vi "Set IC.vi"(8 "error in (no error)":errorcluster, 10 "IC":variant, 11 "IC in":refnum<class "NI_IC.lvclass">) -> (0 "error out":errorcluster, 3 "IC out":refnum<class "NI_IC.lvclass">)   [LabVIEW 2020, in "NI_PDE.lvlib" / "NI_IC.lvclass"]
uses:
  <vilib>/gmath/pde.llb/ICClass/NI_IC.lvclass
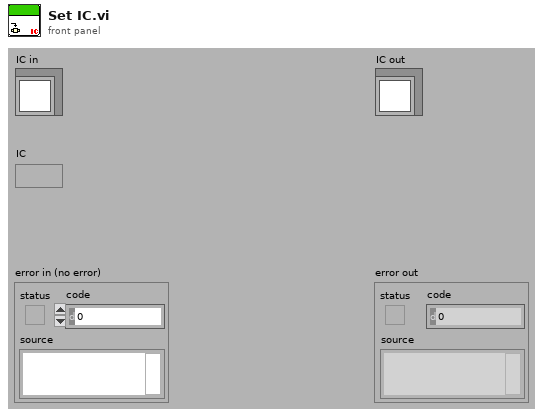
[diagram p1: front panel]
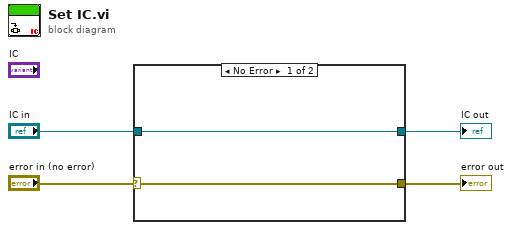
[diagram p0: block diagram]
diagram:
  n1 = case shown="No Error" "error in (no error)" {
    selector: "error in (no error)" -> [w5 w8]
    tunnel: "IC in" -> [w6 w7]
    tunnel: [w6 w7] -> w4
    tunnel: [w5 w8] -> w3
    frame No Error {
    }
    frame Error {
    }
  }
  "IC out" <- w4
  "error out" <- w3
